vi "Init Device.vi"(7 "Layout Ref":refnum<vi>, 8 "error in (no error)":errorcluster, 10 "Chan# Array":i32[](array[numeric]), 11 "Agilent ESG in":refnum<class "Agilent ESG.lvclass">) -> (0 "error out":errorcluster, 3 "Agilent ESG out":refnum<class "Agilent ESG.lvclass">)   [LabVIEW 2013, in "Agilent ESG.lvclass"]
doc: "Initialize the correct columns and their default appearance.\nUse the front panel to change default appearance of the device in the Add/Manage devices.\n\nOpen a specific device implementation for details."
uses:
  Agilent ESG.lvclass
  TypeDefs/ColumnAppearCluster.ctl
  ColumnVIs/Column/Column.lvclass
  Agilent ESG.lvclass/Agilent ESG.ctl
panel:
  in  "Default Display":T2
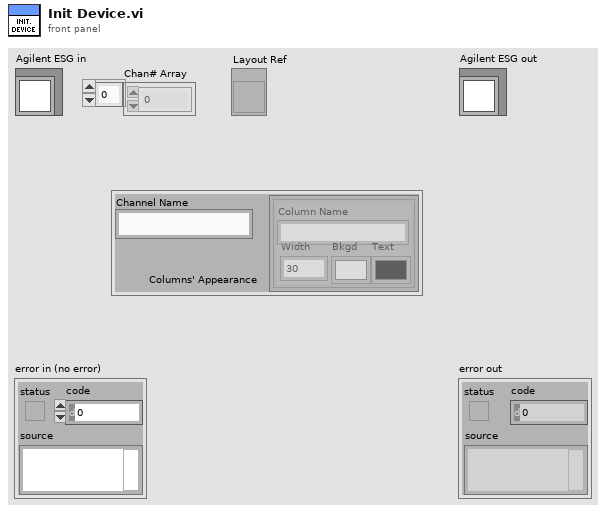
[diagram p1: front panel]
types:
  T1 = typedef "ColumnAppearCluster.ctl" = cluster{"Column Name":string, "Width":u32, "Bkgd":u32[], "Text":u32[]}
  T2 = cluster{"Channel Name":string, "Columns' Appearance":T1[]}
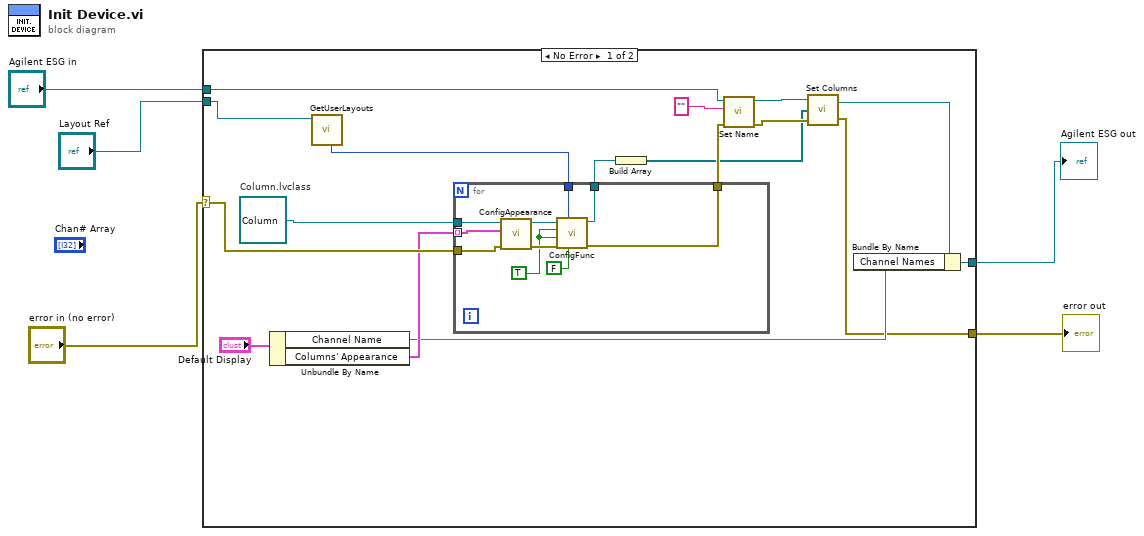
[diagram p0: block diagram]
diagram:
  n1 = case shown="No Error" "error in (no error)" {
    selector: "error in (no error)" -> [w18 w33]
    tunnel: "Layout Ref" -> [w22 _]
    tunnel: "Agilent ESG in" -> [w21 w34]
    tunnel: [w13 w34] -> w2
    tunnel: [w10 w33] -> w1
    frame No Error {
      w7 = refnum<class "Column.lvclass"> refnum  # Column.lvclass
      n2 = Unbundle By Name("Default Display") -> ("Channel Name"=w15:string, "Columns' Appearance"=w16:T1[])
      n3 = call "GetUserLayouts.vi"("Layout Ring Refnum"=w22) -> ("Num User Layouts"=w17:i32)  [unwired: 6 in, 4 out]
      n4 = for {
        tunnel: w7 -> [w32]
        tunnel: w18 -> [w30]
        tunnel: [w27] -> w8
        tunnel: w17 -> [w26]
        tunnel: w16 -> [w25] mode=indexing
        tunnel: [w23] -> w12
        w28 = TRUE ("Disableable? (True)")
        n5 = call "ConfigAppearance.vi"("error in (no error)"=w30, "Column Appearance"=w25, "Column in"=w32) -> ("error out"=w29:errorcluster, "Column out"=w31:refnum<class "Column.lvclass">)  [unwired: 7 in]
        n6 = call "ConfigFunc.vi"("isRampable? (True"=FALSE, "Num Layouts (ignored)"=w26, "error in (no error)"=w29, "isVariable? (True)"=w28, "Disableable? (True)"=w28, "Column in"=w31) -> ("error out"=w23:errorcluster, "Column out"=w27:refnum<class "Column.lvclass">)  [unwired: 4 in]
      }
      n7 = Build Array(w8) -> (w6:refnum<class "Column.lvclass">[])
      n8 = call-dynamic "Set Name.vi"("error in (no error)"=w12, "Name"="", "Device in"=w21) -> ("error out"=w11:errorcluster, "Device out"=w19:refnum<class "Agilent ESG.lvclass">)  [unwired: 7 in]
      n9 = call-dynamic "Set Columns.vi"("error in (no error)"=w11, "Columns"=w6, "Device in"=w19) -> ("error out"=w10:errorcluster, "Device out"=w14:refnum<class "Agilent ESG.lvclass">)  [unwired: 1 in]
      n10 = Bundle By Name(cluster=w14, "Channel Names"=w15) -> (w13:refnum<class "Agilent ESG.lvclass">)
    }
    frame Error {
    }
  }
  "error out" <- w1
  "Agilent ESG out" <- w2
